vi "Trim_Space.vi"() -> ()   [LabVIEW 2019]
panel:
  out "Trim Lenth":i32
  out "Trim Result":string
  out "length":i32
  in  "String":string
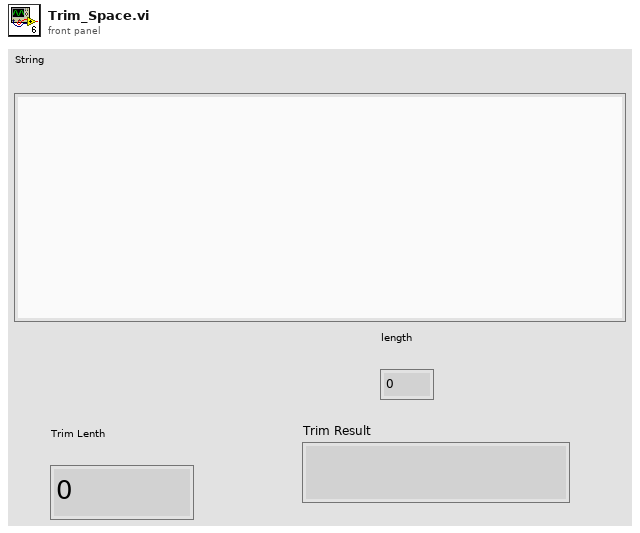
[diagram p1: front panel]
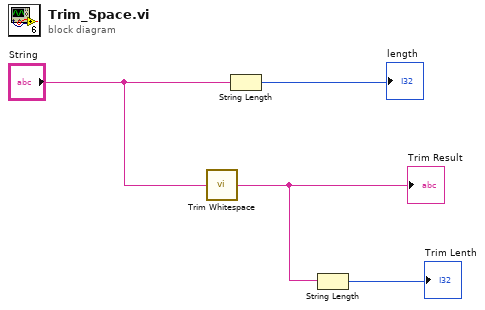
[diagram p0: block diagram]
diagram:
  n1 = call <vilib>:"Trim Whitespace.vi"("string"="String") -> ("trimmed string"=w2:string)  [unwired: 1 in]
  "Trim Result" <- w2
  n2 = String Length(string="String") -> (length=→"length":i32)
  n3 = String Length(string=w2) -> (length=→"Trim Lenth":i32)
